vi "Parse DB.vi"(8 "error in (no error)":errorcluster, 11 "Path in":path=path "C:/work/SE/Opportunities/2012/Pilatus/201210/TestXMLs/Receiver.xml") -> (0 "error out":errorcluster, 3 "channels":T1)   [LabVIEW 2012, in "AIT 429 System Explorer.lvlib"]
uses:
  AIT 429 System Explorer.lvlib
  Controls/AIT_Channel Array.ctl
  Controls/AIT_Channel.ctl
  Controls/AIT_Label.ctl
  Controls/AIT_Word.ctl
  Controls/ARINCParam.ctl
  Shared/Controls and Global/TransferType.ctl
  <userlib>/ARINC-429/vi/enum/Owl429ChannelSpeed.ctl
  <userlib>/ARINC-429/vi/BoardConfig/Owl429_BoardConfig_getChannelDirection.vi
  Parse DB Channel.vi
  <userlib>/ARINC-429/Owl429.lvlib
  ARINC 429 Shared.lvlib
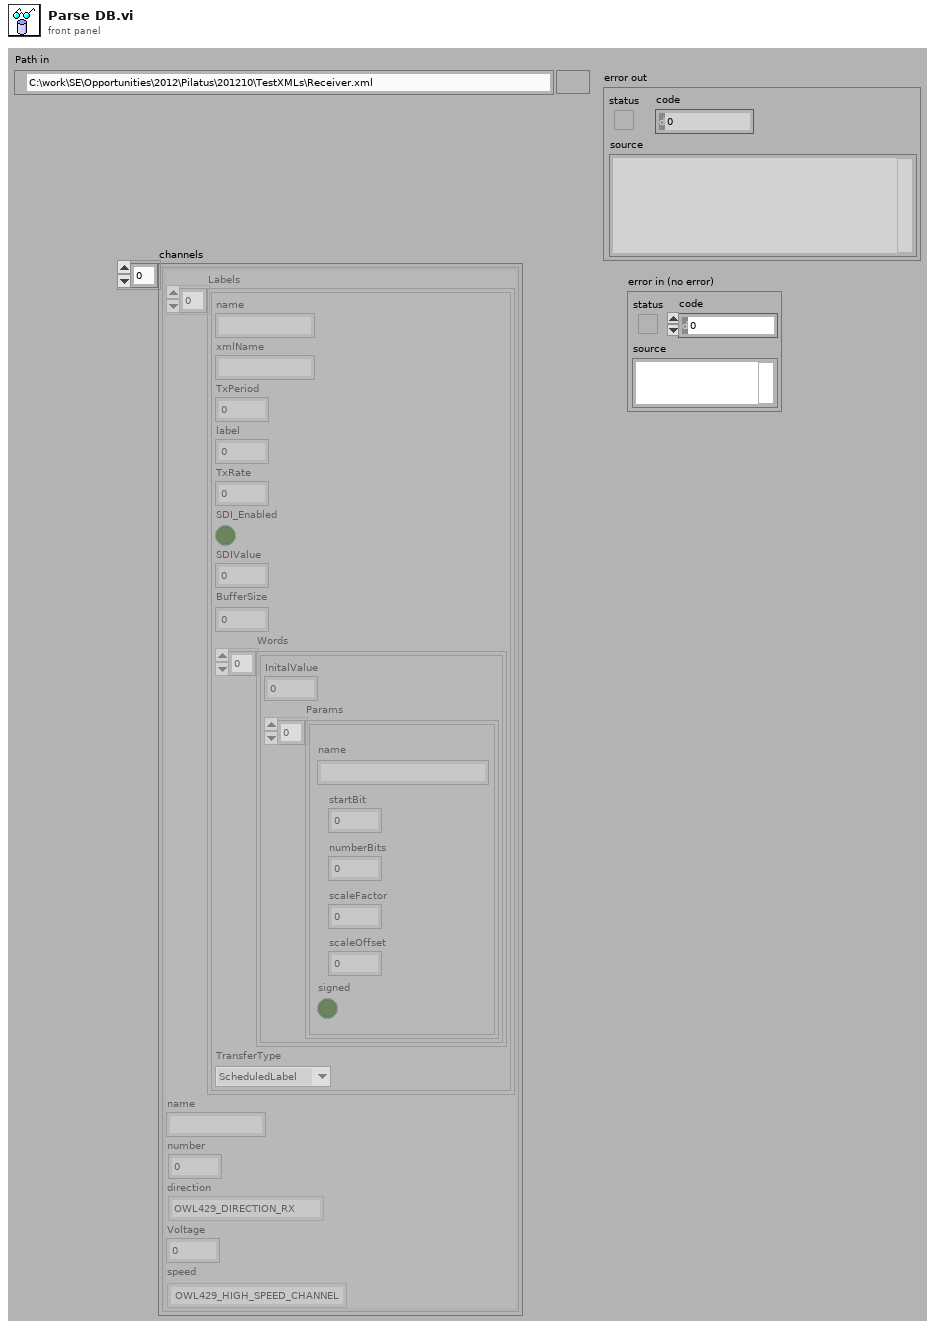
[diagram p1: front panel]
types:
  T1 = typedef "AIT 429 System Explorer.lvlib/AIT_Channel Array.ctl" = T2[]
  T2 = typedef "AIT 429 System Explorer.lvlib/AIT_Channel.ctl" = cluster{"Labels":T3[], "name":string, "number":u8, "direction":enum16{"OWL429_DIRECTION_RX", "OWL429_DIRECTION_TX"}, "Voltage":dbl, "speed":T7}
  T3 = typedef "AIT 429 System Explorer.lvlib/AIT_Label.ctl" = cluster{"name":string, "xmlName":string, "TxPeriod":u32, "label":u32, "TxRate":dbl, "SDI_Enabled":bool, "SDIValue":u8, "BufferSize":u32, "Words":T4[], "TransferType":T6}
  T4 = typedef "AIT 429 System Explorer.lvlib/AIT_Word.ctl" = cluster{"InitalValue":u32, "Params":T5[]}
  T5 = typedef "AIT 429 System Explorer.lvlib/ARINCParam.ctl" = cluster{"name":string, "startBit":i32, "numberBits":i32, "scaleFactor":dbl, "scaleOffset":dbl, "signed":bool}
  T6 = typedef "ARINC 429 Shared.lvlib/TransferType.ctl" = enum16{"ScheduledLabel", "Acyclic", "Block", "Strobe"}
  T7 = typedef "Owl429.lvlib/Owl429ChannelSpeed.ctl" = enum16{"OWL429_HIGH_SPEED_CHANNEL", "OWL429_LOW_SPEED_CHANNEL"}
  T8 = typedef "AIT 429 System Explorer.lvlib/ChannelParams.ctl" = cluster{"ChannelNum":u8, "LabelParams":T9[], "direction":enum16{"OWL429_DIRECTION_RX", "OWL429_DIRECTION_TX"}}
  T9 = typedef "AIT 429 System Explorer.lvlib/LabelParam.ctl" = cluster{"LabelInfo":T10, "ARINCParams":T5[]}
  T10 = typedef "AIT 429 System Explorer.lvlib/LabelInfo.ctl" = cluster{"label":u32, "SDI_Enabled":bool, "SDI":u8}
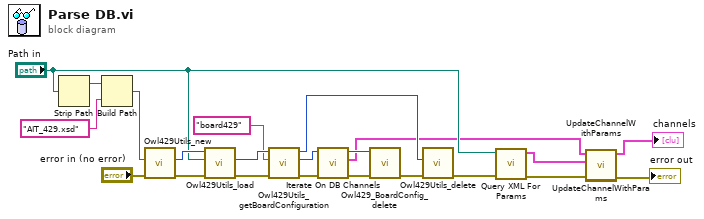
[diagram p0: block diagram]
diagram:
  n1 = Strip Path(path="Path in") -> (stripped path=w11:path)  [unwired: 1 out]
  n2 = Build Path(base path=w11, name or relative path="AIT_429.xsd") -> (appended path=w21:path)
  n3 = call <userlib>:"Owl429Utils_new.vi"("error in (no error)"="error in (no error)", "Xml Schema Path in"=w21) -> ("error out"=w20:errorcluster, "xml config handle"=w19:u32)  [unwired: 8 in]
  n4 = call <userlib>:"Owl429Utils_load.vi"("error in (no error)"=w20, "Path in"="Path in", "xml config handle"=w19) -> ("error out"=w9:errorcluster, "xml config handle"=w18:u32)  [unwired: 7 in]
  n5 = call <userlib>:"Owl429Utils_getBoardConfiguration.vi"("error in (no error)"=w9, "X Path"="board429", "xml config handle"=w18) -> ("error out"=w13:errorcluster, "board config handle"=w12:u32, "xml config handle"=w16:u32)  [unwired: 6 in]
  n6 = call "Iterate On DB Channels.vi"("error out"=w13, "board config handle"=w12) -> ("error IO"=w8:errorcluster, "channels"=w4:T1, "board config handle"=w14:u32)  [unwired: 7 in]
  n7 = call <userlib>:"Owl429_BoardConfig_delete.vi"("error in (no error)"=w8, "config handle"=w14) -> ("error out"=w17:errorcluster)  [unwired: 9 in]
  n8 = call <userlib>:"Owl429Utils_delete.vi"("error in (no error)"=w17, "xml config handle"=w16) -> ("error out"=w7:errorcluster)  [unwired: 9 in]
  n9 = call "Query XML For Params.vi"("error in (no error)"=w7, "XML File Path"="Path in") -> ("error out"=w2:errorcluster, "Array"=w3:T8[])  [unwired: 8 in]
  n10 = call "UpdateChannelWithParams.vi"("error in"=w2, "ParamArray"=w3, "channels in"=w4) -> ("error out"=→"error out":errorcluster, "channels out"=→"channels":T1)  [unwired: 7 in]
  n11 = call "UpdateChannelWithParams.vi"() -> ()  [unwired: 10 in, 2 out]
